vi "Update Nodes.vi"(8 "error in (no error)":errorcluster, 11 "Debug GUI Module in":refnum<class "Debug GUI Module.lvclass">) -> (0 "error out":errorcluster, 3 "Debug GUI Module out":refnum<class "Debug GUI Module.lvclass">)   [LabVIEW 2020, in "VolatusGUI.lvlib" / "Debug GUI Module.lvclass"]
uses:
  Debug GUI Module.lvclass
  C:/dev/lv20CE/relink/lv-volatus/Volatus/Module/Module.lvclass
  Volatus/Module/Module.lvclass/Module.ctl
  Debug GUI Module.lvclass/Debug GUI Module.ctl
  <vilib>/httpClient/LabVIEWHTTPClient.lvlib
  Volatus/DebugHTTPController/DebugHTTPController.lvclass
  Volatus/Module/Module.lvclass
  Volatus/VolatusAPI/VolatusAPI.lvclass
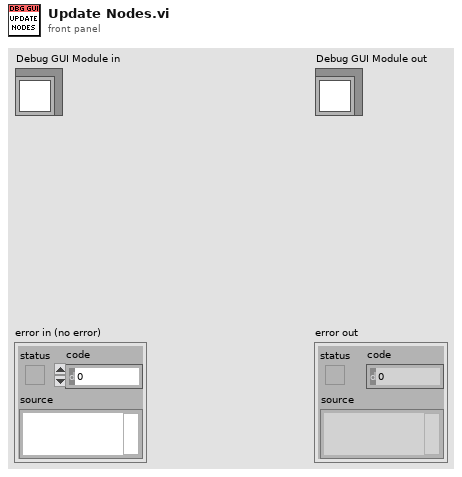
[diagram p1: front panel]
types:
  T1 = typedef "VolatusGUI.lvlib/Debug GUI Module.lvclass/Node Status.ctl" = cluster{"URL":string, "Status Tree":map{string[], T2}}
  T2 = typedef "Volatus.lvlib/Module Status.ctl" = cluster{"Hierarchy":string[], "State":T3, "Substatus":map{string, string}, "Metrics":map{string, dbl}}
  T3 = typedef "Volatus.lvlib/Module.lvclass/State.ctl" = enum16{"Unknown", "Launched", "Starting", "Running", "Stopping", "Stopped", "Error - Starting", "Error - Run", "Error - Stopping"}
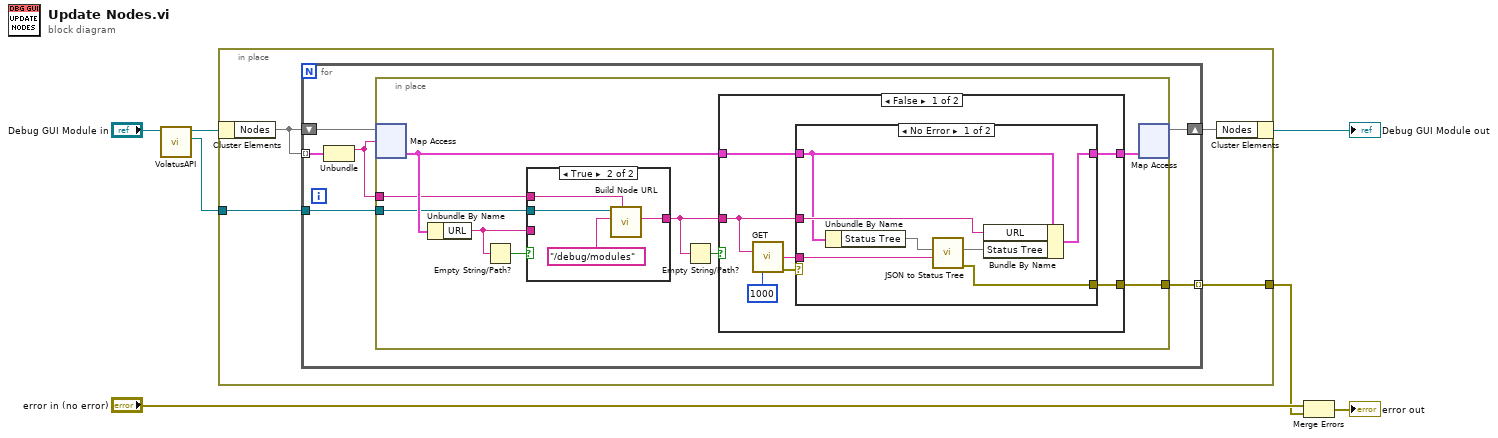
[diagram p0: block diagram]
diagram:
  n1 = call "VolatusAPI.vi"("Module in"="Debug GUI Module in") -> ("VolatusAPI"=w1:refnum<class "VolatusAPI.lvclass">, "Module out"=w2:refnum<class "Debug GUI Module.lvclass">)  [unwired: 9 in]
  n2 = in-place {
    in-place-border: [w9] -> w3
    in-place-border: w1 -> [w8]
    n3 = in-place-cluster #1(w2) -> ("Nodes"=w11:map{string, T1})
    n4 = for {
      shift-right: [w15] -> w10
      shift-left: w11 -> [w16]
      tunnel: w11 -> [w17] mode=indexing
      tunnel: [w14] -> w9 mode=indexing
      tunnel: w8 -> [w13]
      n5 = Unbundle(w17) -> ("Node"=w12:string)  [unwired: 1 out]
      n6 = in-place {
        in-place-border: [w26] -> w14
        in-place-border: w13 -> [w23]
        in-place-border: w12 -> [w22]
        n7 = in-place-map #2(w16, w12) -> (w25:T1)  [unwired: 1 in, 1 out]
        n8 = Unbundle By Name(w25) -> ("URL"=w20:string)
        n9 = Empty String/Path?(string/path=w20) -> (empty?=w21:bool)
        n10 = case shown="True" w21 {
          tunnel: w23 -> [_ w48]
          tunnel: w22 -> [_ w47]
          tunnel: w20 -> [w44 _]
          tunnel: [w44 w45] -> w19
          frame False {
          }
          frame True {
            n11 = call "Build Node URL.vi"("Node Name"=w47, "Path"="/debug/modules", "VolatusAPI in"=w48) -> ("Request URL"=w45:string)  [unwired: 6 in, 2 out]
          }
        }
        n12 = Empty String/Path?(string/path=w19) -> (empty?=w18:bool)
        n13 = case shown="False" w18 {
          tunnel: [w31 _] -> w26
          tunnel: w25 -> [w30 w43]
          tunnel: [w29 w43] -> w24
          tunnel: w19 -> [w28 _]
          frame False {
            n14 = call <vilib>:"GET.vi"("url"=w28, "timeout (10000)"=1000) -> ("body"=w32:string, "error out"=w33:errorcluster)  [unwired: 10 in, 2 out]
            n15 = case shown="No Error" w33 {
              selector: w33 -> [_ w42]
              tunnel: w32 -> [w37 _]
              tunnel: [w40 w42] -> w31
              tunnel: w30 -> [w35 w41]
              tunnel: [w38 w41] -> w29
              tunnel: w28 -> [w36 _]
              frame No Error {
                n16 = Unbundle By Name(w35) -> ("Status Tree"=w34:map{string[], T2})
                n17 = call "JSON to Status Tree.vi"("JSON"=w37, "Status Tree in"=w34) -> ("error out"=w40:errorcluster, "Status Tree"=w39:map{string[], T2})  [unwired: 8 in]
                n18 = Bundle By Name(cluster=w35, "URL"=w36, "Status Tree"=w39) -> (w38:T1)
              }
              frame Error {
              }
            }
          }
          frame True {
          }
        }
        n19 = in-place-map #2(w24) -> (w15:map{string, T1})  [unwired: 1 in, 2 out]
      }
    }
    n20 = in-place-cluster #1("Nodes"=w10) -> (→"Debug GUI Module out":refnum<class "Debug GUI Module.lvclass">)
  }
  n21 = Merge Errors("error in (no error)", w3) -> (→"error out":errorcluster)
